vi "MainEmail.vi"() -> ()   [LabVIEW 2020]
uses:
  EmailField/Write CorrectColorBG.vi
  EmailField/Write CorrectColorText.vi
  EmailField/Write ErrorColorBG.vi
  EmailField/Write ErrorColorText.vi
  EmailField/EmailField.lvclass
panel:
  in  "EmailField":string
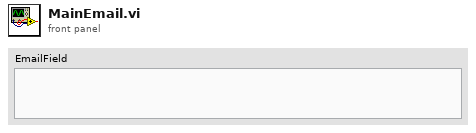
[diagram p1: front panel]
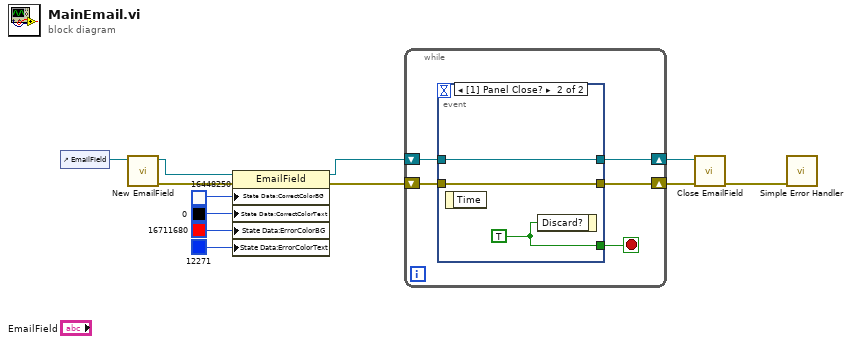
[diagram p0: block diagram]
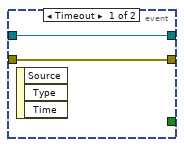
[diagram p2: hidden frame]
diagram:
  n1 = control-ref of="EmailField"() -> (w11:refnum<vi>)
  n2 = call "New EmailField.vi"("Reference"=w11) -> ("error out"=w12:errorcluster, "EmailField out"=w6:refnum<class "EmailField.lvclass">)  [unwired: 9 in]
  n3 = property class="EmailField"(reference=w6, error in=w12, "State Data:CorrectColorBG"=u32 16448250, "State Data:CorrectColorText"=u32 0, "State Data:ErrorColorBG"=u32 16711680, "State Data:ErrorColorText"=u32 12271) -> (reference out=w5:refnum<class "EmailField.lvclass">, error out=w7:errorcluster)
  n4 = while {
    shift-right: [w16] -> w10
    shift-left: w7 -> [w17]
    shift-right: [w13] -> w8
    shift-left: w5 -> [w14]
    stop <- w15 stop-if-true
    n5 = event shown="[1] Panel Close?" {
      selector: _ -> [_ _]
      dyn-events: _ -> [_ _]
      timeout: _ -> [_ _]
      tunnel: [_ w21] -> w15
      tunnel: w14 -> [w18 w20]
      tunnel: w17 -> [w19 w22]
      tunnel: [w19 w22] -> w16
      tunnel: [w18 w20] -> w13
      event Timeout {
        n6 = event-data() -> ()  [unwired: 1 in, 3 out]
      }
      event Panel Close? {
        w21 = TRUE ("Discard?")
        n7 = event-data() -> ()  [unwired: 1 in, 1 out]
        n8 = event-data("Discard?"=w21) -> ()  [unwired: 1 in, 1 out]
      }
    }
  }
  n9 = call "Close EmailField.vi"("error in (no error)"=w10, "EmailField in"=w8) -> ("error out"=w9:errorcluster)  [unwired: 9 in]
  n10 = call <vilib>:"Simple Error Handler.vi"("error in (no error)"=w9) -> ()  [unwired: 4 in, 5 out]
